vi "Init File Config.vi"(7 "Operation":T1, 8 "error in (no error)":errorcluster, 10 "Path":path) -> (0 "error out":errorcluster, 3 "ConfigFile out":refnum<class "ConfigFile.lvclass">)   [LabVIEW 2017, in "ImportExport.lvlib" / "ConfigFile.lvclass"]
uses:
  ConfigFile.lvclass
  Operation.ctl
  ConfigFile.lvclass/ConfigFile.ctl
  ImportExport.lvlib
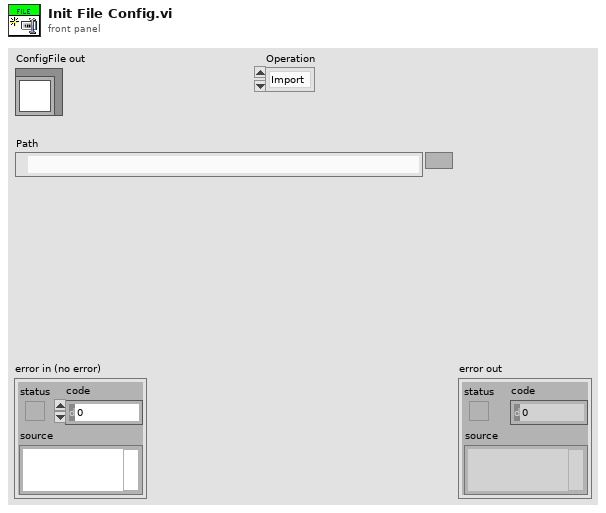
[diagram p1: front panel]
types:
  T1 = typedef "ImportExport.lvlib/Operation.ctl" = enum16{"Import", "Export"}
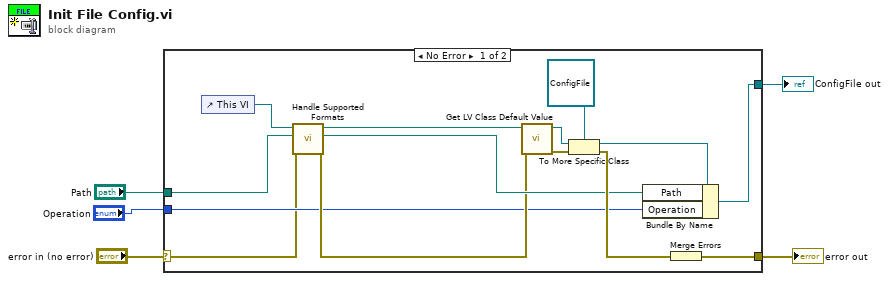
[diagram p0: block diagram]
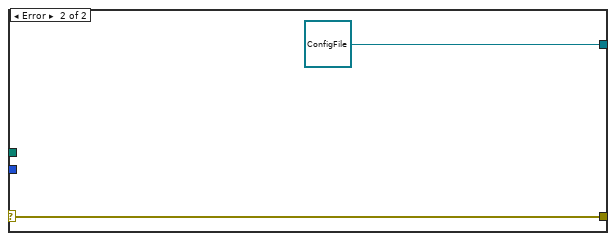
[diagram p2: hidden frame]
diagram:
  n1 = case shown="No Error" "error in (no error)" {
    selector: "error in (no error)" -> [w6 w21]
    tunnel: [w19 w21] -> w4
    tunnel: "Path" -> [w11 _]
    tunnel: [w14 refnum<class "ConfigFile.lvclass"> refnum ("Shared Variables CD 2.0 Configuration.lvlib:ConfigFile.lvclass")] -> w2
    tunnel: "Operation" -> [w7 _]
    frame No Error {
      n2 = control-ref of="This VI"() -> (w12:refnum<vi>)
      n3 = call "Handle Supported Formats.vi"("error in (no error)"=w6, "FilePath"=w11, "VI in"=w12) -> ("error out"=w8:errorcluster, "dup FilePath"=w9:path, "FileType Support Path"=w10:path)  [unwired: 6 in]
      n4 = call <vilib>:"Get LV Class Default Value.vi"("error in (no error)"=w8, "class path"=w10) -> ("error out"=w16:errorcluster, "object"=w17:refnum<class>)  [unwired: 8 in]
      n5 = To More Specific Class(target class=refnum<class "ConfigFile.lvclass"> refnum ("Shared Variables CD 2.0 Configuration.lvlib:ConfigFile.lvclass"), reference=w17, error in=w16) -> (specific class reference=w15:refnum<class "ConfigFile.lvclass">, error out=w13:errorcluster)
      n6 = Bundle By Name(cluster=w15, "Path"=w9, "Operation"=w7) -> (w14:refnum<class "ConfigFile.lvclass">)
      n7 = Merge Errors(w13) -> (w19:errorcluster)
    }
    frame Error {
    }
  }
  "error out" <- w4
  "ConfigFile out" <- w2
